vi "Write Append Numeric.vi"(10 "Append Numeric":u32, 11 "StringIncrement":refnum<class "StringIncrement.Alphabetical.lvclass">) -> (3 "StringIncrement out":refnum<class "StringIncrement.Alphabetical.lvclass">)   [LabVIEW 2014, in "StringIncrement.Alphabetical.lvclass"]
uses:
  StringIncrement.Alphabetical.lvclass
  StringIncrement.Alphabetical.lvclass/StringIncrement.Alphabetical.ctl
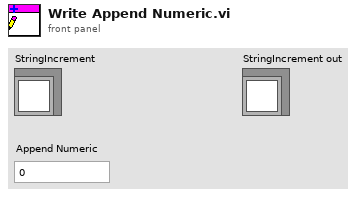
[diagram p1: front panel]
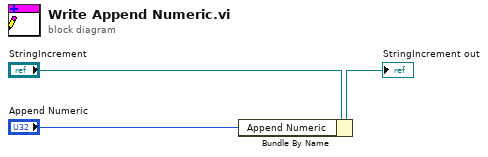
[diagram p0: block diagram]
diagram:
  n1 = Bundle By Name(cluster="StringIncrement", "Append Numeric"="Append Numeric") -> (→"StringIncrement out":refnum<class "StringIncrement.Alphabetical.lvclass">)
